vi "Convert Detection Ball to AI Ball.vi"(5 "fps":dbl, 7 "Lado":enum16{"Esquerdo", "Direito"}(ring) caption="Enum", 11 "Input":T2[](array[typedef])) -> (3 "Output":T1[](array[typedef]))   [LabVIEW 2017]
uses:
  SSL Detection Ball.ctl
  <vilib>/Analysis/Matrix/Datatypes/RealMatrix.ctl
  AI Ball.ctl
  <vilib>/Analysis/Matrix/NI_Matrix.lvlib
panel:
  out "Vel X":dbl
  out "Vel Y":dbl
  in  "fc":dbl=10.0
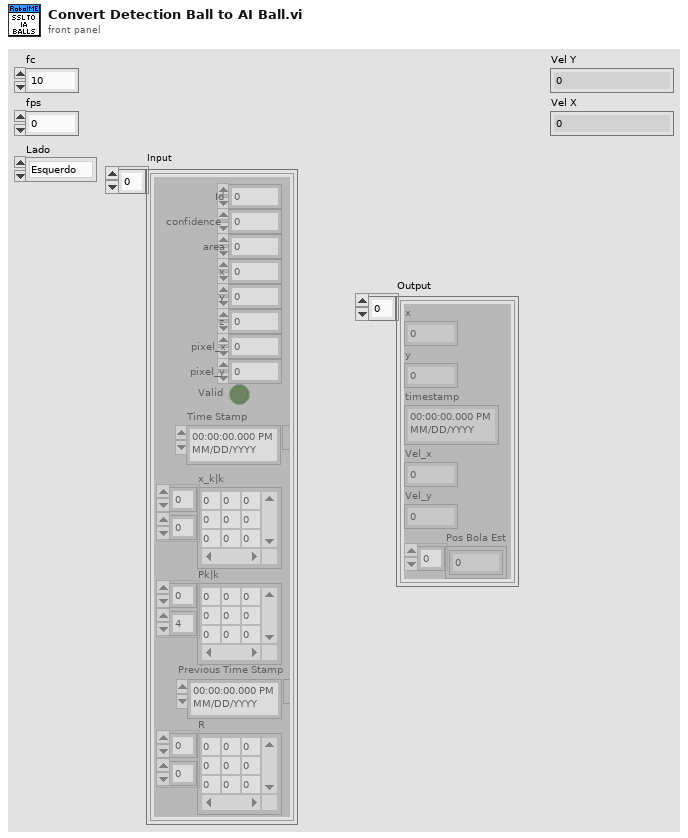
[diagram p1: front panel]
types:
  T1 = typedef "AI Ball.ctl" = cluster{"x":dbl, "y":dbl, "timestamp":timestamp, "Vel_x":dbl, "Vel_y":dbl, "Pos Bola Est":dbl[]}
  T2 = typedef "SSL Detection Ball.ctl" = cluster{"x":sgl, "area":u32, "confidence":sgl, "y":sgl, "z":sgl, "pixel_x":sgl, "pixel_y":sgl, "Valid":bool, "Time Stamp":timestamp, "x_k|k":T3, "Pk|k":T3, "Id":u32, "Previous Time Stamp":timestamp, "R":T3}
  T3 = typedef "NI_Matrix.lvlib/RealMatrix.ctl" = dbl[][]
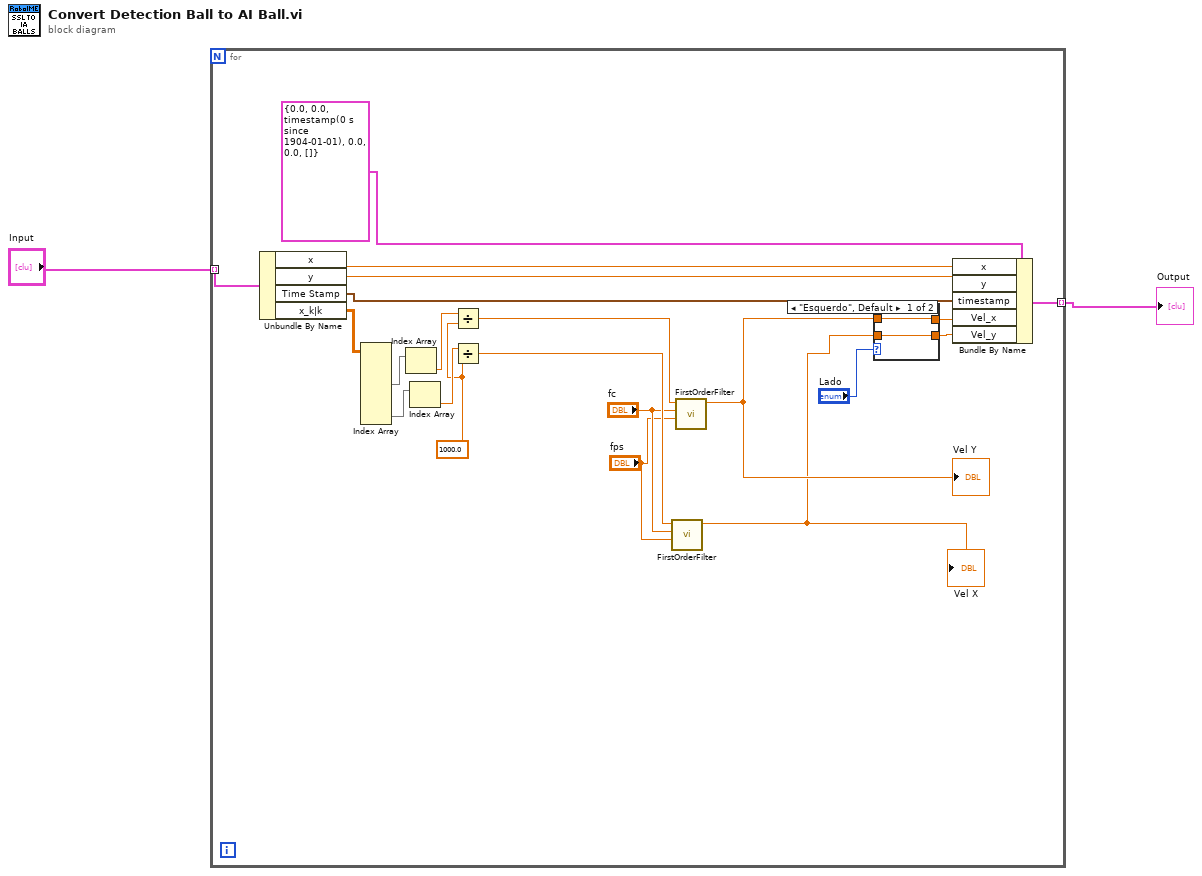
[diagram p0: block diagram]
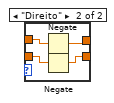
[diagram p2: hidden frame]
diagram:
  n1 = for {
    tunnel: "Input" -> [w22] mode=indexing
    tunnel: [w20] -> w1 mode=indexing
    w12 = 1000.0
    n2 = Unbundle By Name(w22) -> ("x"=w21:sgl, "y"=w18:sgl, "Time Stamp"=w19:timestamp, "x_k|k"=w17:T3)
    n3 = Index Array(array=w17) -> (element #2=w16:dbl[], element #4=w15:dbl[])  [unwired: 8 in, 2 out]
    n4 = Index Array(array=w16) -> (element=w14:dbl)  [unwired: 1 in]
    n5 = Index Array(array=w15) -> (element=w13:dbl)  [unwired: 1 in]
    n6 = Divide(x=w14, y=w12) -> (x/y=w8:dbl)
    n7 = Divide(x=w13, y=w12) -> (x/y=w6:dbl)
    n8 = call "FirstOrderFilter.vi"("fps"="fps", "fc"="fc", "Numeric in"=w6) -> ("Numeric out"=w5:dbl)  [unwired: 8 in]
    "Vel X" <- w5
    n9 = call "FirstOrderFilter.vi"("fps"="fps", "fc"="fc", "Numeric in"=w8) -> ("Numeric out"=w7:dbl)  [unwired: 8 in]
    "Vel Y" <- w7
    n10 = case shown="\"Esquerdo\", Default" "Lado" {
      tunnel: [w25 w29] -> w10
      tunnel: w7 -> [w25 w28]
      tunnel: [w24 w26] -> w9
      tunnel: w5 -> [w24 w27]
      frame "Esquerdo", Default {
      }
      frame "Direito" {
        n11 = Negate(x=w28) -> (-x=w29:dbl)
        n12 = Negate(x=w27) -> (-x=w26:dbl)
      }
    }
    n13 = Bundle By Name(cluster=T1 {"x"=0.0, "y"=0.0, "timestamp"=timestamp(0 s since 1904-01-01), "Vel_x"=0.0, "Vel_y"=0.0, "Pos Bola Est"=[]} ("Ball"), "x"=w21, "y"=w18, "timestamp"=w19, "Vel_x"=w10, "Vel_y"=w9) -> (w20:T1)
  }
  "Output" <- w1
